vi "WildBugChilGru.vi"() -> ()   [LabVIEW 2014]
uses:
  <vilib>/Utility/miscctls.llb/LVPointTypeDef.ctl
  <vilib>/Utility/miscctls.llb/LVBoundsTypeDef.ctl
  <vilib>/Utility/miscctls.llb/LVPositionTypeDef.ctl
  <vilib>/Utility/xml.llb/Read From XML File(string).vi
  <vilib>/Utility/xml.llb/Write to XML File(string).vi
  <vilib>/Instr/_visa.llb/VISA Configure Serial Port (Instr).vi
  <vilib>/Analysis/3filter.llb/IIR Filter (DBL).vi
  <vilib>/gmath/NI_Gmath.lvlib
  <vilib>/Analysis/NI_AALBase.lvlib
panel:
  out "XY-Graph":cluster{dbl[], dbl[]}[](graph)
  in  "Registerkarte":T1(tab)
  in  "Zündung [Imp/U]":dbl=1.0
  in  "Übersetzung ermitteln aus":T2(ring)
  in  "Getriebe [1:]":dbl=4.0
  in  "Reifenumfang [m]":dbl=1.2
  in  "Dauer [s]":dbl=5.0
  in  "nKuWe/nRolle":dbl=1.0 format="%#.3f"
  in  "Lufttemperatur [°C]":dbl
  in  "Luftfeuchtigkeit [%]":dbl=43.8
  in  "Luftdruck [mbar]":dbl=1013.45
  in  "Messung Klimadaten":bool=TRUE
  in  "Gleitender Mittelwert":u8=35
  in  "Differenzenquotient":u8=12
  in  "n vom Gas [1/min]":dbl=5000.0
  in  "Rollengeber [Inkr/U]":u16=200
  in  "Rollenumfang [m]":dbl=0.613
  in  "Rollenträgheit [kgm²]":dbl=0.402
  in  "Recalc":bool
  in  "Leistung":bool=TRUE caption="Messung Klimadaten"
  in  "Ende":bool
  out "Datenspeicher":T3={"Fahrzeugdaten"="", "date/time string"="", "Rolle [Inkr/U]"=200, "Rollenumfang [m]"=0.613, "Rollenträgheit [kgm²]"=0.402, "Zündung [Imp/U]"=1.0, "Getriebe [1:]"=4.0, "Reifenumfang [m] "=1.2, "element"=0.0, "Gl. Mittelwert"=35, "Differenzenquotient"=12, "Polynom"=0, "dT [s]"=0.0, "element"=0.0, "Lufttemperatur [°C]"=0.0, "Luftfeuchtigkeit [%]"=43.8, "Luftdruck [mbar]"=1013.45, [], [], "Best Polynomial Fit"=[], [], "Übersetzung ermitteln aus"=0, "[s]"=5.0, "nmin [1/min]"=0.0, "nmax [1/min]"=0.0, "n vom Gas [1/min]"=5000.0, "dT-Array [s]"=[], [], "Boolesch"=TRUE, "Serielle Schnittstelle"="COM6", "nKuWe/nRolle"=1.0}
  out "COM-Fehlerrate":string="0 / 0,0%"
  in  "Konfiguration:":bool
  in  "Speichern":bool
  in  "Drucken":bool
  out "Pmax":string="0,0 PS"
  out "Ergebnis":string
  in  "Fahrzeugdaten":string
  out "Untersetzung\nermittelt":bool
  out "Untersetzung":dbl format="%#.3f"
  in  "Start":bool
  out "Füllstand Lesepuffer":u64(slide)=1 scale=1.0..100.0
  out "Hinterrad\n[km/h]":dbl(knob) step=5.0 scale=0.0..150.0
  out "Welle\n[1/min]":cluster{dbl, dbl}(knob) scale=0.0..14000.0
  out "Lesepuffer":string="\n"
  in  "Serielle Schnittstelle":refnum<visa-resource-name>="COM6"
  out "Untersetzung-Graph":dbl(graph)=198.99999999999997 caption="Untersetzung"
  # "1. n konstant halten\n2. START\n3. n weiter halten\n4. bei GO: Vollgas\n5. vom Gas gehen"
  # "Live-Tacho"
  # "Zündung\nRolle"
  # "Untersetzung aus:"
  # "Eingabe <> Messen"
  # "Tacho <> Leistung"
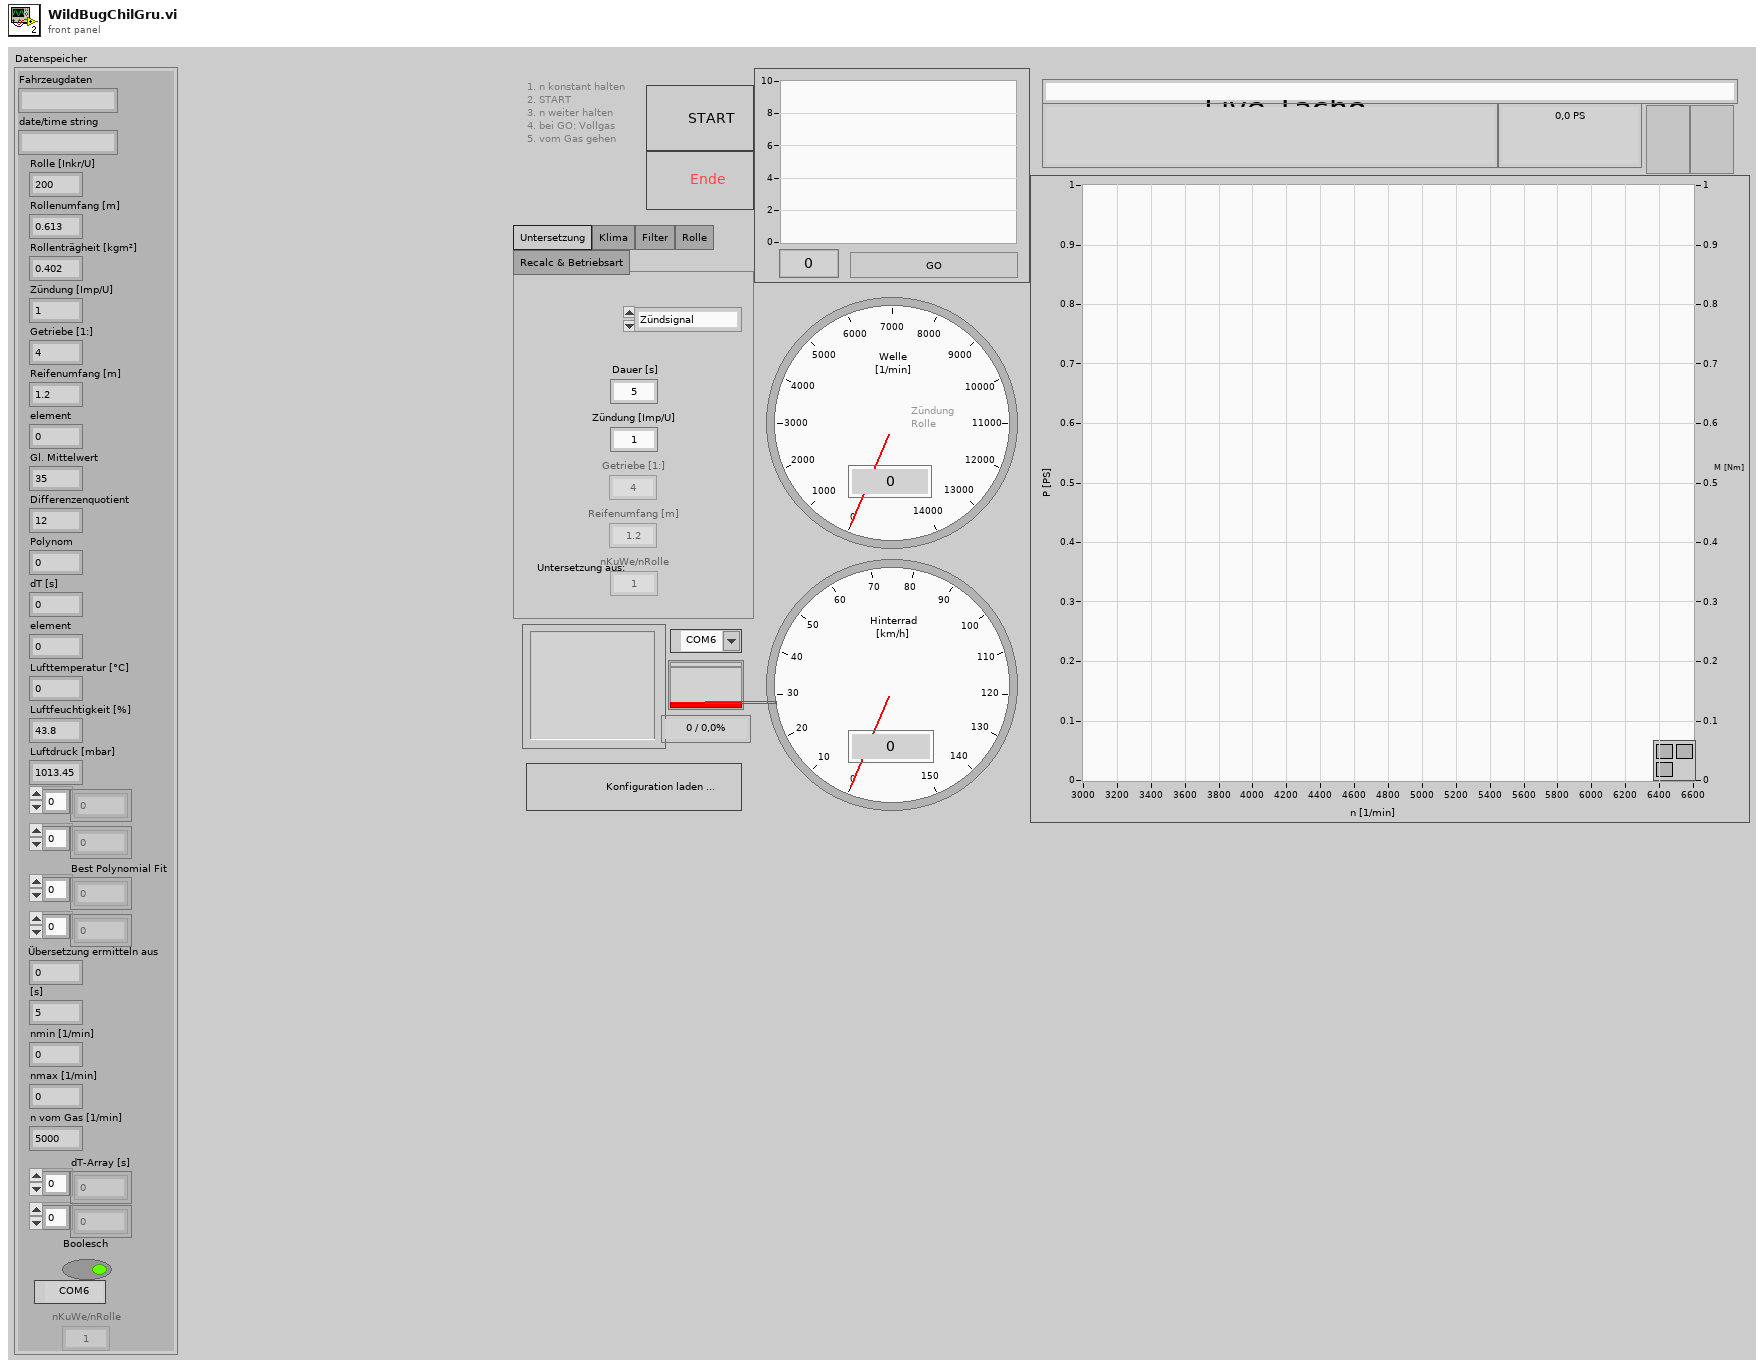
[diagram p1: front panel]
types:
  T1 = enum32{"Untersetzung", "Klima", "Filter", "Rolle", "Recalc & Betriebsart"}
  T2 = enum8{"Zündsignal", "Getriebe & Reifen", "nKuWe / nRolle"}
  T3 = cluster{"Fahrzeugdaten":string, "date/time string":string, "Rolle [Inkr/U]":u16, "Rollenumfang [m]":dbl, "Rollenträgheit [kgm²]":dbl, "Zündung [Imp/U]":dbl, "Getriebe [1:]":dbl, "Reifenumfang [m] ":dbl, "element":dbl, "Gl. Mittelwert":u8, "Differenzenquotient":u8, "Polynom":u8, "dT [s]":dbl, "element":dbl, "Lufttemperatur [°C]":dbl, "Luftfeuchtigkeit [%]":dbl, "Luftdruck [mbar]":dbl, dbl[], dbl[], "Best Polynomial Fit":dbl[], dbl[], "Übersetzung ermitteln aus":u8, "[s]":dbl, "nmin [1/min]":dbl, "nmax [1/min]":dbl, "n vom Gas [1/min]":dbl, "dT-Array [s]":dbl[], i32[], "Boolesch":bool, "Serielle Schnittstelle":refnum<visa-resource-name>, "nKuWe/nRolle":dbl}
  T4 = enum8{"Enabled", "Disabled", "Disabled and Grayed Out"}
  T5 = cluster{"Fahrzeugdaten":string, "date/time string":string, "Rollengeber [Inkr/U]":u16, "Rollenumfang [m]":dbl, "Rollenträgheit [kgm²]":dbl, "Zündung [Imp/U]":dbl, "Getriebe [1:]":dbl, "Reifenumfang [m] ":dbl, "mean value":dbl, "Gleitender Mittelwert":u8, "Differenzenquotient":u8, i32, dbl, "element":dbl, "Lufttemperatur [°C]":dbl, "Luftfeuchtigkeit [%]":dbl, "Luftdruck [mbar]":dbl, dbl[], dbl[], dbl[], dbl[], "Übersetzung ermitteln aus":enum8{"Zündsignal", "Getriebe & Reifen", "nKuWe / nRolle"}, "Dauer [s]":dbl, dbl, dbl, "n vom Gas [1/min]":dbl, dbl[], i32[], "Messung Klimadaten":bool, "VISA resource name out":refnum<visa-resource-name>, "nKuWe/nRolle":dbl}
  T6 = cluster{"Fahrzeugdaten":string, "date/time string":string, "Rolle [Inkr/U]":u16, "Rollenumfang [m]":dbl, "Rollenträgheit [kgm²]":dbl, "Zündung [Imp/U]":dbl, "Getriebe [1:]":dbl, "Reifenumfang [m] ":dbl, "element":dbl, "Gl. Mittelwert":u8, "Differenzenquotient":u8, "Polynom":u8, "element":dbl, "element":dbl, "Lufttemperatur [°C]":dbl, "Luftfeuchtigkeit [%]":dbl, "Luftdruck [mbar]":dbl, dbl[], dbl[], "Best Polynomial Fit":dbl[], dbl[], "Übersetzung ermitteln aus":u8, "[s]":dbl, "nmin [1/min]":dbl, "nmax [1/min]":dbl, "n vom Gas [1/min]":dbl, dbl[], i32[], "Boolesch":bool, "Serielle Schnittstelle":refnum<visa-resource-name>, dbl}
  T7 = typedef "LVPointTypeDef.ctl" = cluster{"Horizontal":i16, "Vertical":i16}
  T8 = typedef "LVPositionTypeDef.ctl" = cluster{"Left":i32, "Top":i32}
  T9 = typedef "LVBoundsTypeDef.ctl" = cluster{"Width":u32, "Height":u32}
  T10 = enum16{"Left Button", "Center Button", "Right Button", "Window Close"}
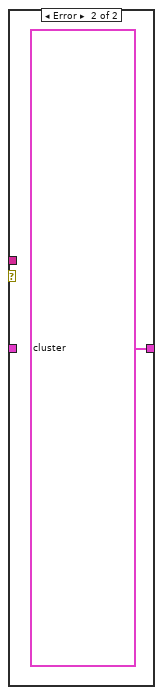
[diagram p2: hidden frame]
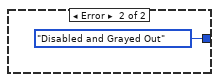
[diagram p3: hidden frame]
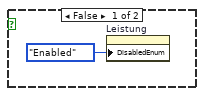
[diagram p4: hidden frame]
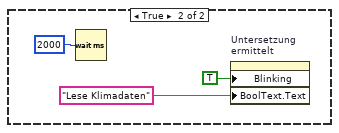
[diagram p5: hidden frame]
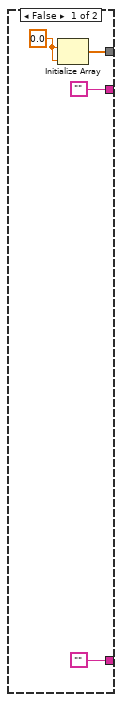
[diagram p8: hidden frame]
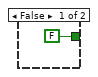
[diagram p9: hidden frame]
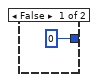
[diagram p11: hidden frame]
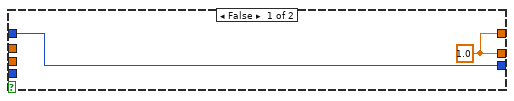
[diagram p13: hidden frame]
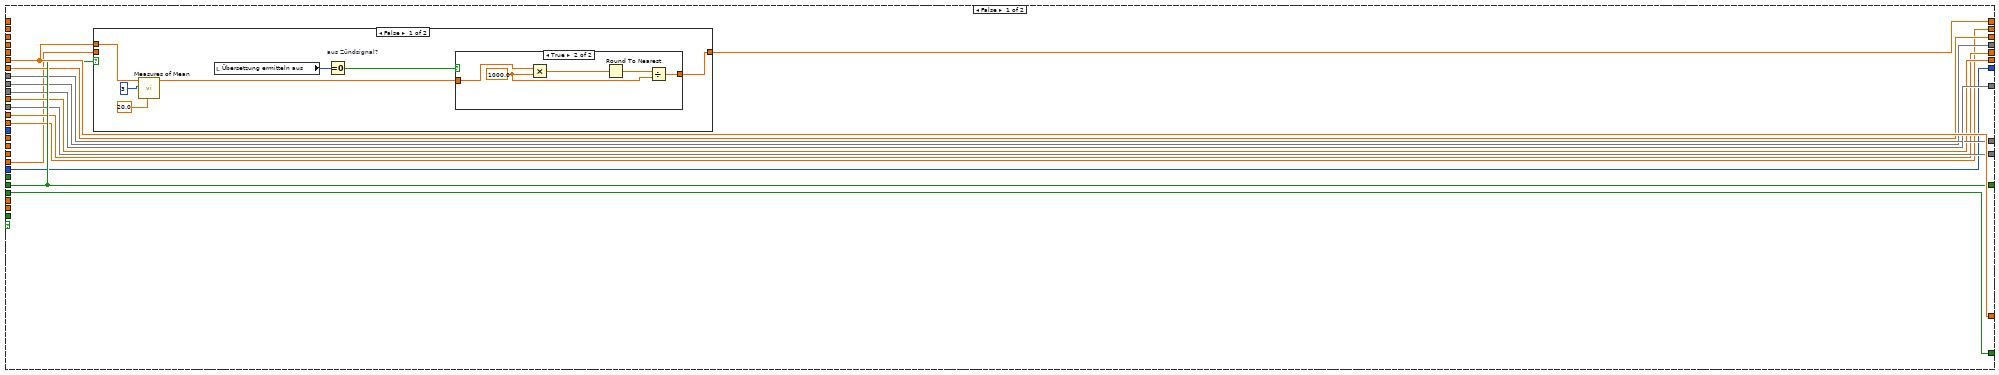
[diagram p14: hidden frame]
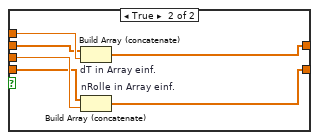
[diagram p17: hidden frame]
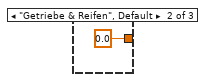
[diagram p20: hidden frame]
diagram:
  n1 = while {
    stop <- w1 stop-if-true
    n2 = local read "Start"() -> (w2:bool)
    n3 = case shown="True" w2 {
      frame False {
        n4 = property on="Leistung" class="Bool. (strikt)"("DisabledEnum"=T4."Enabled" ("Deaktiviert")) -> ()  [unwired: 2 in, 2 out]
      }
      frame True {
        n5 = flat-sequence {
          tunnel: [w137] -> w123
          tunnel: [w136] -> w122
          tunnel: [w134] -> w121
          tunnel: ["Leistung"] -> w8
          tunnel: w123 -> [w148]
          tunnel: w122 -> [w152]
          tunnel: [0] -> w120
          tunnel: [1.0 ("element")] -> w119
          tunnel: [w150] -> w118
          tunnel: [w162] -> w117
          tunnel: [0] -> w116
          tunnel: [w150] -> w115
          tunnel: [-5] -> w114
          tunnel: [w159] -> w113
          tunnel: [w157] -> w112
          tunnel: [w156] -> w111
          tunnel: [0.0] -> w110
          tunnel: [w148] -> w109
          tunnel: [w152] -> w108
          tunnel: w121 -> [w151]
          tunnel: [w151] -> w107
          tunnel: w8 -> [w147]
          tunnel: [w147] -> w4
          tunnel: w120 -> [w189]
          tunnel: [w189] -> w106
          tunnel: w119 -> [w188]
          tunnel: [w188] -> w105
          tunnel: w118 -> [w187]
          tunnel: [w187] -> w104
          tunnel: w117 -> [w186]
          tunnel: [w186] -> w103
          tunnel: w116 -> [w185]
          tunnel: [w185] -> w102
          tunnel: w115 -> [w184]
          tunnel: [w184] -> w101
          tunnel: w114 -> [w183]
          tunnel: [w183] -> w100
          tunnel: w113 -> [w182]
          tunnel: [w182] -> w99
          tunnel: w112 -> [w181]
          tunnel: [w181] -> w98
          tunnel: w111 -> [w180]
          tunnel: [w180] -> w97
          tunnel: w110 -> [w179]
          tunnel: [w179] -> w96
          tunnel: w109 -> [w178]
          tunnel: [w175] -> w95
          tunnel: w108 -> [w177]
          tunnel: [w176] -> w94
          tunnel: w107 -> [w174]
          tunnel: [w174] -> w10
          tunnel: [w173] -> w5
          tunnel: w4 -> [w173]
          tunnel: w106 -> [w214]
          tunnel: [w214] -> w93
          tunnel: w105 -> [w213]
          tunnel: [w213] -> w92
          tunnel: w104 -> [w212]
          tunnel: [w212] -> w91
          tunnel: w103 -> [w211]
          tunnel: [w211] -> w90
          tunnel: w102 -> [w210]
          tunnel: [w210] -> w89
          tunnel: w101 -> [w209]
          tunnel: [w209] -> w88
          tunnel: w100 -> [w208]
          tunnel: [w208] -> w87
          tunnel: w99 -> [w207]
          tunnel: [w207] -> w86
          tunnel: w98 -> [w206]
          tunnel: [w206] -> w85
          tunnel: w97 -> [w205]
          tunnel: [w205] -> w84
          tunnel: w96 -> [w204]
          tunnel: [w204] -> w83
          tunnel: w95 -> [w203]
          tunnel: [w203] -> w82
          tunnel: w94 -> [w202]
          tunnel: [w202] -> w81
          tunnel: [w200] -> w11
          tunnel: w10 -> [w200]
          tunnel: [w199] -> w6
          tunnel: w5 -> [w199]
          tunnel: w93 -> [w231]
          tunnel: [w231] -> w80
          tunnel: w92 -> [w230]
          tunnel: [w230] -> w79
          tunnel: w91 -> [w229]
          tunnel: [w229] -> w78
          tunnel: w90 -> [w228]
          tunnel: [w228] -> w77
          tunnel: w89 -> [w227]
          tunnel: [w227] -> w76
          tunnel: w88 -> [w226]
          tunnel: [w226] -> w75
          tunnel: w87 -> [w225]
          tunnel: [w225] -> w74
          tunnel: w86 -> [w224]
          tunnel: [w224] -> w73
          tunnel: w85 -> [w223]
          tunnel: [w223] -> w72
          tunnel: w84 -> [w222]
          tunnel: [w222] -> w71
          tunnel: w83 -> [w221]
          tunnel: [w221] -> w70
          tunnel: w82 -> [w220]
          tunnel: [w219] -> w69
          tunnel: w81 -> [w217]
          tunnel: [w218] -> w68
          tunnel: w11 -> [w216]
          tunnel: [w215] -> w7
          tunnel: w6 -> [w215]
          tunnel: w80 -> [w296]
          tunnel: w79 -> [w295]
          tunnel: w78 -> [w294]
          tunnel: w77 -> [w293]
          tunnel: w76 -> [w292]
          tunnel: w75 -> [w291]
          tunnel: w74 -> [w290]
          tunnel: w73 -> [w289]
          tunnel: w72 -> [w288]
          tunnel: w71 -> [w287]
          tunnel: w70 -> [w286]
          tunnel: w69 -> [w267]
          tunnel: [w296] -> w67
          tunnel: [w295] -> w66
          tunnel: [w294] -> w65
          tunnel: [w293] -> w64
          tunnel: [w292] -> w63
          tunnel: [w291] -> w62
          tunnel: [w290] -> w61
          tunnel: [w289] -> w60
          tunnel: [w288] -> w59
          tunnel: [w287] -> w58
          tunnel: [w286] -> w57
          tunnel: [w267] -> w56
          tunnel: [w266] -> w55
          tunnel: [w285] -> w54
          tunnel: [w284] -> w53
          tunnel: [w283] -> w52
          tunnel: ["Gleitender Mittelwert"] -> w51
          tunnel: w68 -> [w266]
          tunnel: [w261] -> w14
          tunnel: [w260] -> w13
          tunnel: [w259] -> w9
          tunnel: w7 -> [w259]
          tunnel: [w305] -> w23
          tunnel: [w306] -> w24
          tunnel: [w307] -> w25
          tunnel: [w308] -> w26
          tunnel: [w299] -> w21
          tunnel: [w298] -> w22
          tunnel: [w309] -> w27
          tunnel: [w310] -> w28
          tunnel: [w311] -> w30
          tunnel: [w312] -> _
          tunnel: [w313] -> w32
          tunnel: [w314] -> w33
          tunnel: [w315] -> w46
          tunnel: [w316] -> w12
          tunnel: [w317] -> w48
          tunnel: [w318] -> w49
          tunnel: [w319] -> w50
          tunnel: w67 -> [w319]
          tunnel: w66 -> [w318]
          tunnel: w65 -> [w317]
          tunnel: w64 -> [w316]
          tunnel: w63 -> [w315]
          tunnel: w62 -> [w314]
          tunnel: w61 -> [w313]
          tunnel: w60 -> [w312]
          tunnel: w59 -> [w311]
          tunnel: w58 -> [w310]
          tunnel: w57 -> [w309]
          tunnel: w56 -> [w301]
          tunnel: w55 -> [w300]
          tunnel: w54 -> [w308]
          tunnel: w53 -> [w307]
          tunnel: w52 -> [w306]
          tunnel: w51 -> [w305]
          frame #0 {
            w142 = u16 0 items=["None", "XON/XOFF", "RTS/CTS", "XON/XOFF & RTS/CTS", "DTR/DSR", "XON/XOFF & DTR/DSR"] ("flow control (0:none)")
            w143 = u16 10 items=["1.0"=10, "1.5"=15, "2.0"=20] ("stop bits (10: 1 bit)")
            w135 = FALSE  # Enable Termination Char (T)
            w138 = u32 10000  # timeout (10sec)
            n6 = call-poly "VISA Configure Serial Port"("VISA resource name"="Serielle Schnittstelle", "timeout (10sec)"=w138, "Enable Termination\nChar (T)"=w135, "baud rate (9600)"=u32 115200 ("baudrate (250000)"), "data bits (8)"=u16 8, "parity (0:none)"=enum16{"None", "Odd", "Even", "Mark", "Space"}."None", "stop bits (10: 1 bit)"=w143, "flow control (0:none)"=w142) -> ("VISA resource name out"=w140:refnum<visa-resource-name>, "error out"=w139:errorcluster)  [unwired: 6 in]
            n7 = And(x="Messung Klimadaten", y="Leistung") -> (x .and. y?=w134:bool)
            n8 = VISA Clear(VISA resource name=w140, error in (no error)=w139) -> (VISA resource name out=w137:refnum<visa-resource-name>, error out=w136:errorcluster)
          }
          frame #1 {
            w149 = T4."Disabled and Grayed Out" ("Deaktiviert")
            w155 = 0.0  # Graphen löschen
            w158 = 0
            w163 = 0.0
            w150 = FALSE
            w156 = ""
            n9 = case shown="False" w151 {
              frame False {
                n10 = property on="Untersetzung\nermittelt" class="Bool. (strikt)"("Blinking"=TRUE ("Blinkend"), "BoolText.Text"="Initialisiere" ("Beschriftung.Text")) -> ()  [unwired: 2 in, 2 out]
              }
              frame True {
                n11 = Wait (ms)(milliseconds to wait=u32 2000 ("Zu wartende ms")) -> ()  [unwired: 1 out]
                n12 = property on="Untersetzung\nermittelt" class="Bool. (strikt)"("Blinking"=TRUE ("Blinkend"), "BoolText.Text"="Lese Klimadaten" ("Beschriftung.Text")) -> ()  [unwired: 2 in, 2 out]
              }
            }
            n13 = Build Array(w155) -> (w154:dbl[])
            n14 = property on="Drucken" class="Bool. (strikt)"("DisabledEnum"=w149) -> ()  [unwired: 2 in, 2 out]
            n15 = property on="Übersetzung ermitteln aus" class="Enum (strikt)"("DisabledEnum"=w149) -> ()  [unwired: 2 in, 2 out]
            n16 = property on="Konfiguration:" class="Bool. (strikt)"("DisabledEnum"=w149) -> ()  [unwired: 2 in, 2 out]
            n17 = property on="Ende" class="Bool. (strikt)"("DisabledEnum"=w149) -> ()  [unwired: 2 in, 2 out]
            n18 = property on="Leistung" class="Bool. (strikt)"("DisabledEnum"=w149) -> ()  [unwired: 2 in, 2 out]
            n19 = property on="Speichern" class="Bool. (strikt)"("DisabledEnum"=w149) -> ()  [unwired: 2 in, 2 out]
            n20 = property on="Untersetzung-Graph" class="SVDiagr (strikt)"("History Data"=w154) -> ()  [unwired: 2 in, 2 out]
            n21 = local write "Pmax"(w156) -> ()
            n22 = local write "COM-Fehlerrate"(w156) -> ()
            n23 = local write "Ergebnis"(w156) -> ()
            n24 = Initialize Array(w158, w158) -> (w157:i32[])
            n25 = Initialize Array(w163, w163) -> (w162:dbl[])
            n26 = Initialize Array(0.0 ("y"), 0) -> (w159:dbl[])
          }
          frame #2 {
            n27 = case shown="True" w174 {
              tunnel: w178 -> [w191 w195]
              tunnel: w177 -> [w190 w194]
              tunnel: [w190 w193] -> w176
              tunnel: [w191 w192] -> w175
              frame False {
              }
              frame True {
                n28 = Concatenate Strings("e" ("String"), "\n") -> (w198:string)
                n29 = VISA Write(VISA resource name=w195, write buffer=w198, error in (no error)=w194) -> (VISA resource name out=w192:refnum<visa-resource-name>, error out=w193:errorcluster)  [unwired: 1 out]
              }
            }
          }
          frame #3 {
            n30 = Wait (ms)(milliseconds to wait=u32 500 ("Zu wartende ms")) -> ()  [unwired: 1 out]
          }
          frame #4 {
            n31 = case shown="True" w216 {
              tunnel: w220 -> [w233 w254]
              tunnel: [w233 w253] -> w219
              tunnel: [w232 w252] -> w218
              tunnel: w217 -> [w232 w251]
              frame False {
              }
              frame True {
                w236 = ";" ("Regulärer Ausdruck")
                n32 = property class="Instr"(reference=w254, error in=w251) -> (reference out=w257:refnum<visa-resource-name>, error out=w256:errorcluster, "Serial Settings:Number of Bytes at Serial Port"=w255:u32)
                n33 = VISA Read(VISA resource name=w257, byte count=w255, error in (no error)=w256) -> (VISA resource name out=w253:refnum<visa-resource-name>, read buffer=w248:string, error out=w252:errorcluster)  [unwired: 1 out]
                n34 = Search and Replace String(replace all?=TRUE ("Alle ersetzen? (F)"), input string=w248, search string="." ("Such-String"), replace string="," ("Ersetzungs-String (\"\")")) -> (result string=w241:string)  [unwired: 4 in, 3 out]
                n35 = Match Pattern(string=w241, regular expression=w236) -> (before substring=w239:string, after substring=w240:string)  [unwired: 1 in, 2 out]
                n36 = Match Pattern(string=w240, regular expression=w236) -> (before substring=w238:string, after substring=w237:string)  [unwired: 1 in, 2 out]
                n37 = Fract/Exp String To Number(string=w239, offset=0 ("Offset")) -> (number=w247:dbl)  [unwired: 2 in, 1 out]
                n38 = local write "Lufttemperatur [°C]"(w247) -> ()
                n39 = Fract/Exp String To Number(string=w238) -> (number=w244:dbl)  [unwired: 3 in, 1 out]
                n40 = Match Pattern(string=w237, regular expression=w236) -> (before substring=w235:string)  [unwired: 1 in, 3 out]
                n41 = Fract/Exp String To Number(string=w235) -> (number=w246:dbl)  [unwired: 3 in, 1 out]
                n42 = Divide(x=w244, y=100.0 ("x")) -> (x/y=w245:dbl)
                n43 = local write "Luftdruck [mbar]"(w245) -> ()
                n44 = local write "Luftfeuchtigkeit [%]"(w246) -> ()
              }
            }
          }
          frame #5 {
            n45 = Wait (ms)(milliseconds to wait=u32 2000 ("Zu wartende ms")) -> ()  [unwired: 1 out]
            n46 = Add(x="Lufttemperatur [°C]", y=273.15) -> (x+y=w279:dbl)
            n47 = Divide ("M_Welle [Nm]")(x=w279, y=293.15) -> (x/y=w277:dbl)
            n48 = Power Of X(1:w277, 2:0.5) -> (0:w274:dbl)
            n49 = Divide ("M_Welle [Nm]")(x=1013.0, y="Luftdruck [mbar]") -> (x/y=w275:dbl)
            n50 = Multiply "Korrekturfaktor DIN 70020"(x=w275, y=w274) -> (x*y=w285:dbl)
            n51 = local read "Differenzenquotient"() -> (w262:u8)
            n52 = Divide(x="Gleitender Mittelwert", y=2) -> (x/y=w271:dbl)
            n53 = Round Toward -Infinity(1:w271) -> (0:w270:dbl)
            n54 = call <vilib>:"Smoothing Filter Coefficients.vi"("shape"=1, "half-width"=w270, "type"=0) -> ("forward coefficients"=w283:dbl[], "reverse coefficients"=w284:dbl[])  [unwired: 6 in, 1 out]
            n55 = call <vilib>:"Smoothing Filter Coefficients.vi"("shape"=0, "half-width"=w262, "type"=0) -> ("forward coefficients"=w260:dbl[], "reverse coefficients"=w261:dbl[])  [unwired: 6 in, 1 out]
          }
          frame #6 {
            n56 = Concatenate Strings("m" ("String"), "\n") -> (w304:string)
            n57 = property on="Untersetzung\nermittelt" class="Bool. (strikt)"("Blinking"=FALSE ("Blinkend")) -> ()  [unwired: 2 in, 2 out]
            n58 = VISA Write(VISA resource name=w301, write buffer=w304, error in (no error)=w300) -> (VISA resource name out=w298:refnum<visa-resource-name>, error out=w299:errorcluster)  [unwired: 1 out]
          }
        }
        n59 = while {
          tunnel: w22 -> [w440]
          tunnel: w21 -> [w439]
          shift-right: [w506] -> _
          shift-left: w28 -> [w455]
          shift-right: [w501] -> _
          shift-left: w27 -> [w505]
          shift-right: [w500] -> _
          shift-left: w27 -> [w504]
          shift-right: [w459] -> _
          shift-left: w27 -> [w503]
          shift-right: [w485] -> _
          shift-left: w50 -> [w502]
          shift-right: [w447] -> w35
          shift-left: w49 -> [_]
          shift-right: [w464] -> w39
          shift-left: w27 -> [w434]
          shift-right: [w429] -> w37
          shift-left: w27 -> [w461]
          shift-right: [w460] -> _
          shift-left: w12 -> [w497]
          shift-right: [w432] -> _
          shift-left: w48 -> [w474]
          shift-right: [w441] -> _
          shift-left: w12 -> [_]
          shift-right: [w446] -> _
          shift-left: w12 -> [_]
          shift-right: [w494] -> w38
          shift-left: w12 -> [w492]
          shift-right: [w493] -> _
          shift-left: w12 -> [w491]
          shift-right: [w480] -> w45
          shift-left: w12 -> [w490]
          shift-right: [w484] -> _
          shift-left: w12 -> [w488]
          shift-right: [w483] -> w15
          shift-left: w12 -> [w489]
          shift-right: [w482] -> w44
          shift-left: w12 -> [w487]
          shift-right: [w481] -> w43
          shift-left: w12 -> [w486]
          tunnel: [w479] -> w47
          shift-right: [w475] -> w42
          shift-left: w46 -> [w477]
          tunnel: [w478] -> w18
          tunnel: ["n vom Gas [1/min]"] -> w41
          tunnel: ["Rollenumfang [m]"] -> w40
          tunnel: ["Rollenumfang [m]"] -> w34
          shift-right: [w471] -> _
          shift-left: w33 -> [w438]
          shift-right: [w465] -> _
          shift-left: w32 -> [w470]
          shift-right: [w466] -> _
          shift-left: w27 -> [w469]
          shift-right: [w467] -> _
          shift-left: w27 -> [w468]
          shift-right: [w437] -> w31
          shift-left: w12 -> [w463]
          shift-right: [w458] -> _
          shift-left: _ -> [w457]
          shift-right: [w462] -> w29
          shift-left: w30 -> [w456]
          tunnel: [w454] -> w19
          tunnel: w26 -> [w447]
          tunnel: w25 -> [w441]
          tunnel: w24 -> [w446]
          tunnel: w23 -> [w445]
          tunnel: w14 -> [w436]
          tunnel: w13 -> [w435]
          tunnel: w9 -> [w428]
          stop <- w479 stop-if-true
          n60 = property class="Instr"(reference=w440, error in=w439) -> (reference out=w450:refnum<visa-resource-name>, error out=w449:errorcluster, "Serial Settings:Number of Bytes at Serial Port"=w452:u32)
          n61 = Greater?(x=w452, y=u32 1 ("min. Bytes")) -> (0:w448:bool)
          n62 = case shown="True" w448 {
            tunnel: w452 -> [_ w512]
            tunnel: [u32 0 ("Bytes at Port") w512] -> w451
            frame False {
            }
            frame True {
            }
          }
          n63 = case shown="1.." w451 {
            selector: w451 -> [_ w798]
            tunnel: [w748 w792] -> w478
            tunnel: [w747 w793] -> w454
            tunnel: [w752 w794] -> w500
            tunnel: [w753 w791] -> w501
            tunnel: w455 -> [w754 w789]
            tunnel: [w754 w787] -> w506
            tunnel: w505 -> [w753 w779]
            tunnel: w504 -> [w752 w778]
            tunnel: [w749 w777] -> w459
            tunnel: w503 -> [w749 w776]
            tunnel: w502 -> [w751 _]
            tunnel: [w751 w759] -> w485
            tunnel: [w750 w765] -> w458
            tunnel: w457 -> [w750 w764]
            tunnel: w450 -> [w747 w756]
            tunnel: w449 -> [w748 w755]
            frame 0, Default {
              # "No data in from serial port - Nothing to do."
            }
            frame 1.. {
              # "Hz Drum"
              n64 = VISA Read(VISA resource name=w756, byte count=w798, error in (no error)=w755) -> (VISA resource name out=w793:refnum<visa-resource-name>, read buffer=w790:string, error out=w792:errorcluster)  [unwired: 1 out]
              n65 = Concatenate Strings(w789, w790) -> (w761:string)
              "Lesepuffer" <- w761
              n66 = Spreadsheet String To Array(delimiter (Tab)="\n" ("regular expression"), format string="%s" ("regular expression"), spreadsheet string=w761, array type (2D Dbl)=string[] [] ("Array 2")) -> (array=w770:string[])
              n67 = Match Pattern(string=w761, regular expression="[\\n]") -> (before substring=w768:string, after substring=w788:string, offset past match=w802:i32)  [unwired: 1 in, 1 out]
              n68 = Array Size(array=w770) -> (size(s)=w774:i32)
              n69 = Match Pattern(string=w768, regular expression="[;]") -> (before substring=w766:string, after substring=w767:string, offset past match=w763:i32)  [unwired: 1 in, 1 out]
              n70 = Subtract "aktuelle Zeilenanzahl"(x=w774, y=1) -> (x-y=w759:i32)
              n71 = property on="Füllstand Lesepuffer" class="Schieber (strikt)"() -> ("Scale.Maximum"=w758:dbl)  [unwired: 2 in, 2 out]
              n72 = Match Pattern(string=w767, regular expression="[;]") -> (before substring=w797:string, after substring=w800:string, offset past match=w785:i32)  [unwired: 1 in, 1 out]
              n73 = Match Pattern(string=w800, regular expression="[;]") -> (before substring=w796:string, after substring=w795:string, offset past match=w783:i32)  [unwired: 1 in, 1 out]
              n74 = Greater Or Equal To 0?(x=w763) -> (x >= 0?=w762:bool)
              n75 = Greater?(x=w759, y=w758) -> (0:w760:bool)
              n76 = Greater Or Equal To 0?(x=w783) -> (x >= 0?=w782:bool)
              n77 = Greater Or Equal To 0?(x=w785) -> (x >= 0?=w784:bool)
              n78 = Greater Or Equal To 0?(x=w802) -> (x >= 0?=w786:bool)
              n79 = Select(t=w759, s=w760, f=w758) -> (s? t:f=w757:dbl)
              n80 = Build Array(w786, w784, w762, w782) -> (w781:bool[])
              n81 = property on="Füllstand Lesepuffer" class="Schieber (strikt)"("Scale.Maximum"=w757) -> ()  [unwired: 2 in, 2 out]
              n82 = And Array Elements(Boolean array=w781) -> (logical AND=w780:bool)
              n83 = case shown="True" w780 {
                tunnel: w797 -> [_ w813]
                tunnel: w796 -> [_ w818]
                tunnel: w795 -> [_ w817]
                tunnel: [w806 w816] -> w794
                tunnel: [w807 w815] -> w791
                tunnel: w788 -> [_ w814]
                tunnel: [w808 w814] -> w787
                tunnel: w761 -> [w808 _]
                tunnel: w779 -> [w807 _]
                tunnel: w778 -> [w806 _]
                tunnel: [w805 w812] -> w777
                tunnel: w776 -> [w805 _]
                tunnel: w766 -> [_ w811]
                tunnel: [w804 w809] -> w765
                tunnel: w764 -> [w804 _]
                frame False {
                }
                frame True {
                  # "Cyclecounter"
                  # "Hz ComLevel"
                  # "ComLevel\nLevel 10 =   6Hz \nLevel 5 =   12Hz \nLevel 4 =   15Hz\nLevel 3 =   20Hz\nLevel 2 =   33Hz\nLevel 1 =   62Hz"
                  # "Hz Drum"
                  # "Hz Engine"
                  # "t4m"
                  n84 = Fract/Exp String To Number(string=w811) -> (number=w810:dbl)  [unwired: 3 in, 1 out]
                  n85 = Fract/Exp String To Number(string=w817) -> (number=w816:dbl)  [unwired: 3 in, 1 out]
                  n86 = Fract/Exp String To Number(string=w813) -> (number=w812:dbl)  [unwired: 3 in, 1 out]
                  n87 = To Long Integer(number=w810) -> (32bit integer=w809:i32)
                  n88 = Fract/Exp String To Number(string=w818) -> (number=w815:dbl)  [unwired: 3 in, 1 out]
                }
              }
            }
          }
          "Füllstand Lesepuffer" <- w485
          n89 = Not Equal?(x=w457, y=w458) -> (x != y?=w442:bool)
          n90 = case shown="True" w442 {
            tunnel: w470 -> [w516 w527]
            tunnel: [w516 w539] -> w465
            tunnel: w469 -> [w515 w538]
            tunnel: [w515 w524] -> w466
            tunnel: w468 -> [w514 w537]
            tunnel: [w514 w525] -> w467
            tunnel: w458 -> [_ w523]
            tunnel: w456 -> [w513 w522]
            tunnel: [w513 w526] -> w462
            frame False {
            }
            frame True {
              n91 = Build Array (concatenate)(w522, w523) -> (w526:i32[])
              n92 = Greater Or Equal To 0?(x=w527) -> (x >= 0?=w528:bool)
              n93 = case shown="True" w528 {
                tunnel: [w540 w551] -> w524
                tunnel: [w540 w552] -> w525
                tunnel: [w541 w543] -> w539
                tunnel: w538 -> [_ w545]
                tunnel: w537 -> [_ w553]
                tunnel: w523 -> [w541 w542]
                tunnel: w527 -> [_ w543]
                frame False {
                  w540 = 1.0
                }
                frame True {
                  w549 = 65536.0
                  n94 = Add(x=w543, y=w545) -> (x+y=w544:dbl)
                  n95 = Divide(x=w544, y=w549) -> (x/y=w554:dbl)
                  n96 = Increment(x=w553) -> (x+1=w552:dbl)
                  n97 = Round Toward -Infinity(1:w554) -> (0:w550:dbl)
                  n98 = Multiply(x=w550, y=w549) -> (x*y=w548:dbl)
                  n99 = Add(x=w548, y=w542) -> (x+y=w547:dbl)
                  n100 = Increment(x=w547) -> (x+1=w546:dbl)
                  n101 = Subtract(x=w546, y=w543) -> (x-y=w551:dbl)
                }
              }
              n102 = Subtract(x=w524, y=w525) -> (x-y=w519:dbl)
              n103 = Decrement(x=w519) -> (x-1=w518:dbl)
              n104 = Max & Min(x=0, y=w518) -> (max(x,y)=w517:dbl)  [unwired: 1 out]
              n105 = Divide(x=w517, y=w524) -> (x/y=w531:dbl)
              n106 = Greater Than 0?(x=w517) -> (x > 0?=w521:bool)
              n107 = Select(t=u32 16711680, s=w521, f=u32 0) -> (s? t:f=w532:u32)
              n108 = Multiply(x=w531, y=100.0) -> (x*y=w529:dbl)
              n109 = property on="COM-Fehlerrate" class="Str"("Text.TextColor"=w532) -> ()  [unwired: 2 in, 2 out]
              n110 = Format Into String(format string="%d / %.1f%%" ("Format-String"), w517, w529) -> (resulting string=→"COM-Fehlerrate":string)  [unwired: 2 in, 1 out]
            }
          }
          n111 = case "Case-Struktur" shown="True" w442 {
            tunnel: w501 -> [w728 w740]
            tunnel: w500 -> [w727 w739]
            tunnel: [w728 w738] -> w499
            tunnel: [w727 w737] -> w498
            tunnel: w459 -> [_ w732]
            tunnel: w434 -> [w726 _]
            tunnel: [w726 w731] -> w464
            tunnel: w461 -> [_ w736]
            tunnel: "Rollenumfang [m]" -> [_ w735]
            frame False {
            }
            frame True {
              w746 = 60.0 ("y")
              n112 = Reciprocal "Abtastzeit [s]"(x=w732) -> (1/x=w731:dbl)
              n113 = Divide "R [1/s]"(x=w739, y="Rollengeber [Inkr/U]") -> (x/y=w745:dbl)
              n114 = Divide(x=w740, y="Zündung [Imp/U]") -> (x/y=w743:dbl)
              n115 = Multiply "nZ gemessen [1/min]"(x=w743, y=w746) -> (x*y=w738:dbl)
              n116 = Multiply "nR [1/min]"(x=w746, y=w745) -> (x*y=w737:dbl)
              n117 = Multiply "nZ berechnet [1/min]"(x=w737, y=w736) -> (x*y=w744:dbl)
              n118 = Multiply "[m/min]"(x=w737, y=w735) -> (x*y=w741:dbl)
              n119 = Multiply "[km/h]"(x=w741, y=0.06) -> (x*y=→"Hinterrad\n[km/h]":dbl)
              n120 = Bundle(w738, w744) -> (→"Welle\n[1/min]":cluster{dbl, dbl})  [unwired: 1 in]
            }
          }
          n121 = case shown="True" w442 {
            tunnel: w499 -> [_ w647]
            tunnel: w498 -> [_ w646]
            tunnel: "Rollenumfang [m]" -> [_ w650]
            tunnel: [w566 w621] -> w429
            tunnel: w461 -> [w555 w621]
            tunnel: w474 -> [w567 w589]
            tunnel: w497 -> [w568 w653]
            tunnel: [w567 w613] -> w432
            tunnel: [w568 w652] -> w460
            tunnel: w441 -> [_ w649]
            tunnel: w446 -> [_ w648]
            tunnel: [w565 w585] -> w494
            tunnel: [w564 w593] -> w493
            tunnel: w492 -> [w565 w645]
            tunnel: w491 -> [w564 _]
            tunnel: w445 -> [_ w602]
            tunnel: [w563 w627] -> w480
            tunnel: w490 -> [w563 _]
            tunnel: [w562 w592] -> w484
            tunnel: w488 -> [w562 _]
            tunnel: [w561 w628] -> w483
            tunnel: w489 -> [w561 _]
            tunnel: [w560 w639] -> w482
            tunnel: w487 -> [w560 _]
            tunnel: [w559 w638] -> w481
            tunnel: w486 -> [w559 _]
            tunnel: w447 -> [_ w631]
            tunnel: w477 -> [w558 w626]
            tunnel: "n vom Gas [1/min]" -> [_ w615]
            tunnel: [w558 w625] -> w475
            tunnel: w474 -> [_ w624]
            tunnel: w438 -> [w557 w620]
            tunnel: [w557 w619] -> w471
            tunnel: w464 -> [_ w618]
            tunnel: [w556 w586] -> w437
            tunnel: w463 -> [w556 w617]
            tunnel: w436 -> [_ w600]
            tunnel: w435 -> [_ w599]
            tunnel: w428 -> [_ w583]
            frame False {
              n122 = case shown="False" w567 {
                tunnel: w568 -> [w575 _]
                tunnel: [w569 w582] -> w566
                tunnel: w555 -> [_ w582]
                frame False {
                  n123 = call <vilib>:"Measures of Mean.vi"("percent (trim)"=20.0, "type"=3, "x array"=w575) -> ("mean value"=w570:dbl)  [unwired: 7 in, 1 out]
                  n124 = local read "Übersetzung ermitteln aus"() -> (w572:T2)
                  n125 = Equal To 0? "aus Zündsignal?"(x=w572) -> (x = 0?=w571:bool)
                  n126 = case shown="True" w571 {
                    tunnel: w570 -> [w576 w581]
                    tunnel: [w576 w577] -> w569
                    frame False {
                    }
                    frame True {
                      w578 = 1000.0
                      n127 = Multiply(x=w581, y=w578) -> (x*y=w580:dbl)
                      n128 = Round To Nearest(number=w580) -> (nearest integer value=w579:dbl)
                      n129 = Divide(x=w579, y=w578) -> (x/y=w577:dbl)
                    }
                  }
                }
                frame True {
                }
              }
            }
            frame True {
              w634 = 0.00135962  # [W] in [PS]
              w641 = 0.10471975511965978  # 2*Pi/60
              n130 = Not(x=w589) -> (.not. x?=w588:bool)
              n131 = Or(x=w583, y=w588) -> (x .or. y?=w587:bool)
              n132 = local read "Übersetzung ermitteln aus"() -> (w590:T2)
              n133 = case shown="False" w587 {
                tunnel: w646 -> [_ w661]
                tunnel: w645 -> [w654 w660]
                tunnel: w618 -> [_ w659]
                tunnel: w617 -> [w655 w658]
                tunnel: [w654 w657] -> w585
                tunnel: [w655 w656] -> w586
                frame False {
                }
                frame True {
                  n134 = Build Array (concatenate) "dT in Array einf."(w658, w659) -> (w656:dbl[])
                  n135 = Build Array (concatenate) "nRolle in Array einf."(w660, w661) -> (w657:dbl[])
                }
              }
              n136 = local read "Differenzenquotient"() -> (w598:u8)
              n137 = case shown="\"Zündsignal\"" w590 {
                tunnel: w647 -> [_ _ w725]
                tunnel: w646 -> [_ _ w724]
                tunnel: [w720 "nKuWe/nRolle" w723] -> w651
                tunnel: w650 -> [w721 _ _]
                frame "Getriebe & Reifen" {
                  n138 = Divide(x=w721, y="Reifenumfang [m]") -> (x/y=w719:dbl)
                  n139 = Multiply(x=w719, y="Getriebe [1:]") -> (x*y=w720:dbl)
                }
                frame "nKuWe / nRolle" {
                }
                frame "Zündsignal" {
                  n140 = Divide(x=w725, y=w724) -> (x/y=w723:dbl)
                }
              }
              n141 = Multiply(x=2, y=w598) -> (x*y=w596:i32)
              n142 = Increment(x=w596) -> (x+1=w594:i32)
              n143 = Index Array(array=w586, index=1 ("Index")) -> (element=w605:dbl)
              n144 = Index Array(array=w585, index=1 ("Index")) -> (element=w611:dbl)
              n145 = Initialize Array(w605, w594) -> (w603:dbl[])
              n146 = Initialize Array(w611, w602) -> (w610:dbl[])
              n147 = Insert Into Array(array=w586, index=0 ("Index"), new element=w603) -> (w601:dbl[])
              n148 = Insert Into Array(array=w585, index=0 ("Index"), new element=w610) -> (w608:dbl[])
              n149 = call-poly <vilib>:"IIR Filter.vi"("Forward Coefficients"=w599, "Reverse Coefficients"=w600, "X"=w601) -> ("Filtered X"=w595:dbl[])  [unwired: 1 in, 1 out]
              n150 = call-poly <vilib>:"IIR Filter.vi"("Forward Coefficients"=w648, "Reverse Coefficients"=w649, "X"=w608) -> ("Filtered X"=w607:dbl[])  [unwired: 1 in, 1 out]
              n151 = case shown="False" w589 {
                selector: w589 -> [_ w716]
                tunnel: w651 -> [w704 _]
                tunnel: w653 -> [w706 w715]
                tunnel: [w701 w716] -> w644
                tunnel: [w705 w715] -> w652
                tunnel: w620 -> [w703 w714]
                tunnel: [w701 w714] -> w619
                tunnel: w590 -> [w700 _]
                frame False {
                  n152 = Build Array (concatenate)(w706, w704) -> (w705:dbl[])
                  n153 = case shown="\"Zündsignal\"" w700 {
                    tunnel: ["Dauer [s]" 0.0 ("Dauer [s]") 0.0] -> w702
                    frame "Zündsignal" {
                      n154 = property on="Untersetzung\nermittelt" class="Bool. (strikt)"("Blinking"=TRUE ("Blinkend"), "BoolText.Text"="Ermittle Übersetzung" ("Boolescher Text.Text")) -> ()  [unwired: 2 in, 2 out]
                    }
                    frame "Getriebe & Reifen", Default {
                    }
                    frame "nKuWe / nRolle" {
                    }
                  }
                  n155 = call "Verstrichene Zeit"("Time Target (s)"=w702, "Reset"=w703) -> ("Time has Elapsed"=w701:bool)  [unwired: 10 in, 7 out]
                  n156 = case shown="True" w701 {
                    frame False {
                    }
                    frame True {
                      n157 = property on="Untersetzung\nermittelt" class="Bool. (strikt)"("Blinking"=FALSE ("Blinkend"), "BoolText.Text"="Go" ("Boolescher Text.Text")) -> ()  [unwired: 2 in, 2 out]
                    }
                  }
                  "Untersetzung-Graph" <- w704
                }
                frame True {
                }
              }
              n158 = Array Subset "dT gefiltert [s]"(array=w595, index=w594) -> (w591:dbl[])  [unwired: 1 in]
              n159 = Array Subset "Rolle gefiltert [1/min]"(array=w607, index=w602) -> (w593:dbl[])  [unwired: 1 in]
              n160 = Array Size "Array-Größe"(array=w593) -> (size(s)=w642:i32)
              n161 = Greater?(x=w642, y=w602) -> (0:w643:bool)
              n162 = Square(x=w621) -> (x^2=w640:dbl)
              n163 = Multiply(x=w593, y=w621) -> (x*y=w627:dbl[])
              n164 = Multiply(x=w627, y=w641) -> (x*y=w592:dbl[])
              n165 = Divide(x="Rollenträgheit [kgm²]", y=w640) -> (x/y=w632:dbl)
              n166 = Multiply(x=w632, y=w631) -> (x*y=w630:dbl)
              n167 = And(x=w644, y=w643) -> (x .and. y?=w613:bool)
              n168 = Array Size "Array-Größe"(array=w592) -> (size(s)=w584:i32)
              n169 = Decrement(x=w584) -> (x-1=w629:i32)
              n170 = Select(t=w615, s=w613, f=1000000.0) -> (s? t:f=w616:dbl)
              n171 = Initialize Array(0.0 ("y"), 0) -> (w635:dbl[])
              n172 = for {
                N: w584 -> [_]
                tunnel: "Differenzenquotient" -> [w676]
                tunnel: w592 -> [w684]
                tunnel: w629 -> [w675]
                shift-right: [w681] -> w628
                shift-left: w635 -> [w682]
                tunnel: w627 -> [w679] mode=indexing
                tunnel: w626 -> [w668]
                tunnel: w616 -> [w678]
                tunnel: [w669] -> w625
                tunnel: w624 -> [w667]
                tunnel: w591 -> [w664] mode=indexing
                i -> [w665]
                stop <- w662 stop-if-true
                n173 = Multiply(x=w664, y=2.0) -> (x*y=w666:dbl)
                n174 = Subtract(x=w675, y=w676) -> (x-y=w677:i32)
                n175 = Subtract(x=w665, y=w676) -> (x-y=w697:i32)
                n176 = Add(x=w665, y=w676) -> (x+y=w691:i32)
                n177 = Greater Or Equal?(x=w665, y=w676) -> (x >= y?=w672:bool)
                n178 = Greater?(x=w679, y=w678) -> (0:w680:bool)
                n179 = Max & Min(x=w675, y=w691) -> (min(x,y)=w692:i32)  [unwired: 1 out]
                n180 = Max & Min(x=w697, y=0) -> (max(x,y)=w695:i32)  [unwired: 1 out]
                n181 = Subtract(x=w692, y=w665) -> (x-y=w693:i32)
                n182 = Less Or Equal?(x=w665, y=w677) -> (x <= y?=w673:bool)
                n183 = Subtract(x=w665, y=w695) -> (x-y=w694:i32)
                n184 = Max & Min(x=w694, y=w693) -> (min(x,y)=w685:i32)  [unwired: 1 out]
                n185 = Add(x=w665, y=w685) -> (x+y=w690:i32)
                n186 = Subtract(x=w665, y=w685) -> (x-y=w689:i32)
                n187 = Multiply(x=w685, y=w666) -> (x*y=w683:dbl)
                n188 = Index Array(array=w684, index=w690) -> (element=w687:dbl)
                n189 = Index Array(array=w684, index=w689) -> (element=w688:dbl)
                n190 = Subtract(x=w687, y=w688) -> (x-y=w686:dbl)
                n191 = Divide(x=w686, y=w683) -> (x/y=w674:dbl)
                n192 = Less Than 0?(x=w674) -> (x < 0?=w671:bool)
                n193 = Less Or Equal To 0?(x=w668) -> (x <= 0?=w670:bool)
                n194 = Build Array (concatenate)(w682, w674) -> (w681:dbl[])
                n195 = Compound Arithmetic op=AND(w671, w680, w670, w672, w673, w667) -> (w662:bool)
                n196 = case shown="False" w662 {
                  tunnel: w665 -> [_ w699]
                  tunnel: [w698 w699] -> w669
                  tunnel: w668 -> [w698 _]
                  frame False {
                  }
                  frame True {
                  }
                }
              }
              n197 = Multiply(x=w628, y=w630) -> (x*y=w639:dbl[])
              n198 = Multiply(x=w592, y=w639) -> (x*y=w633:dbl[])
              n199 = Multiply(x=w634, y=w633) -> (x*y=w638:dbl[])
            }
          }
          "Untersetzung\nermittelt" <- w432
          n200 = local read "Übersetzung ermitteln aus"() -> (w433:T2)
          n201 = Equal To 0? "aus Zündsignal?"(x=w433) -> (x = 0?=w431:bool)
          n202 = case shown="True" w428 {
            tunnel: [FALSE w509] -> w476
            tunnel: w475 -> [_ w508]
            frame False {
            }
            frame True {
              n203 = Greater Than 0?(x=w508) -> (x > 0?=w509:bool)
            }
          }
          n204 = And(x=w432, y=w431) -> (x .and. y?=w430:bool)
          n205 = Select(t=w429, s=w432, f=0.0) -> (s? t:f=→"Untersetzung":dbl)
          n206 = case shown="True" w430 {
            tunnel: w429 -> [_ w510]
            frame False {
            }
            frame True {
              n207 = local write "nKuWe/nRolle"(w510) -> ()
            }
          }
          n208 = local read "Start"() -> (w444:bool)
          n209 = Not(x=w444) -> (.not. x?=w443:bool)
          n210 = Or(x=w476, y=w443) -> (x .or. y?=w479:bool)
        }
        n211 = VISA Clear(VISA resource name=w19, error in (no error)=w18) -> (VISA resource name out=w16:refnum<visa-resource-name>, error out=w20:errorcluster)
        n212 = VISA Close(VISA resource name=w16, error in (no error)=w20) -> ()  [unwired: 1 out]
        n213 = case shown="True" w47 {
          tunnel: w45 -> [_ w406]
          tunnel: w44 -> [_ w411]
          tunnel: w43 -> [_ w410]
          tunnel: w42 -> [_ w382]
          tunnel: w15 -> [_ w407]
          tunnel: w41 -> [_ w405]
          tunnel: w40 -> [_ w399]
          tunnel: w35 -> [_ w385]
          tunnel: ["" w384] -> w36
          tunnel: w37 -> [_ w383]
          tunnel: ["" w381] -> _
          tunnel: [w361 w369] -> _
          frame False {
            w362 = 0.0
            n214 = Initialize Array(w362, w362) -> (w361:dbl[])
          }
          frame True {
            w380 = 0
            n215 = Array Subset "P"(array=w410, length=w382) -> (w402:dbl[])  [unwired: 1 in]
            n216 = Array Subset "n"(array=w406, length=w382) -> (w404:dbl[])  [unwired: 1 in]
            n217 = Array Subset "alpha"(array=w407, length=w382) -> (w408:dbl[])  [unwired: 1 in]
            n218 = Array Subset "M"(array=w411, length=w382) -> (w403:dbl[])  [unwired: 1 in]
            n219 = property on="Pmax" class="Str"("Text.FontSize"=48) -> ()  [unwired: 2 in, 2 out]
            n220 = property on="Ergebnis" class="Str"("Text.FontSize"=18) -> ()  [unwired: 2 in, 2 out]
            n221 = Array Size(array=w408) -> (size(s)=w409:i32)
            n222 = for {
              N: w409 -> [w427]
              tunnel: w407 -> [w424]
              tunnel: w406 -> [w421]
              tunnel: w405 -> [w418]
              tunnel: [w416] -> w379
              i -> [w422]
              stop <- w417 stop-if-true
              n223 = Decrement(x=w427) -> (x-1=w426:i32)
              n224 = Subtract(x=w426, y=w422) -> (x-y=w416:i32)
              n225 = Index Array(array=w421, index=w416) -> (element=w420:dbl)
              n226 = Index Array(array=w424, index=w416) -> (element=w425:dbl)
              n227 = Less?(x=w420, y=w418) -> (x < y?=w419:bool)
              n228 = Less Or Equal To 0?(x=w425) -> (x <= 0?=w423:bool)
              n229 = And(x=w423, y=w419) -> (x .and. y?=w417:bool)
            }
            n230 = Increment(x=w379) -> (x+1=w378:i32)
            n231 = Array Subset "P"(array=w402, index=w378) -> (w370:dbl[])  [unwired: 1 in]
            n232 = Array Subset "n"(array=w404, index=w378) -> (w375:dbl[])  [unwired: 1 in]
            n233 = Array Subset "M"(array=w403, index=w378) -> (w369:dbl[])  [unwired: 1 in]
            n234 = Array Max & Min "nmax [1/min]"(array=w375) -> (max value=w401:dbl)  [unwired: 3 out]
            n235 = Array Max & Min "Mmax"(array=w369) -> (max value=w376:dbl, max index (indices)=w372:i32)  [unwired: 2 out]
            n236 = Bundle(w375, w370) -> (w374:cluster{dbl[], dbl[]})  [unwired: 1 in]
            n237 = Bundle(w375, w369) -> (w373:cluster{dbl[], dbl[]})  [unwired: 1 in]
            n238 = Array Max & Min "Pmax"(array=w370) -> (max value=w377:dbl, max index (indices)=w371:i32)  [unwired: 2 out]
            n239 = Index Array "n(Mmax)"(array=w375, index=w372) -> (element=w392:dbl)
            n240 = Index Array "n(Pmax)"(array=w375, index=w371) -> (element=w397:dbl)
            n241 = Multiply(x=w377, y=1.2) -> (x*y=w366:dbl)
            n242 = Multiply(x=w376, y=1.8) -> (x*y=w367:dbl)
            n243 = Divide(x=w401, y=w383) -> (x/y=w400:dbl)
            n244 = Round To Nearest(number=w366) -> (nearest integer value=w365:dbl)
            n245 = Round To Nearest(number=w367) -> (nearest integer value=w368:dbl)
            n246 = Format Into String(format string="%.1f PS" ("Format-String"), w377) -> (resulting string=→"Pmax":string)  [unwired: 2 in, 1 out]
            n247 = Build Array(w374, w373) -> (→"XY-Graph":cluster{dbl[], dbl[]}[])
            n248 = local read "Lufttemperatur [°C]"() -> (w394:dbl)
            n249 = local read "Luftfeuchtigkeit [%]"() -> (w395:dbl)
            n250 = property on="XY-Graph" class="XYGraph (strikt)"("ActYScl"=w380, "YScale.Maximum"=w365, "YScale.Minimum"=w380) -> ()  [unwired: 2 in, 2 out]
            n251 = local read "Luftdruck [mbar]"() -> (w396:dbl)
            n252 = property on="XY-Graph" class="XYGraph (strikt)"("ActYScl"=1, "YScale.Maximum"=w368, "YScale.Minimum"=w380) -> ()  [unwired: 2 in, 2 out]
            n253 = Compound Arithmetic op=MULTIPLY "vmax"(w400, w399, 0.06) -> (w391:dbl)
            n254 = Format Date/Time String(time format string (%c)="%x %H:%M ") -> (date/time string=w384:string)  [unwired: 2 in]
            n255 = Format Into String(format string="%.1f PS bei %d 1/min   |   %.1f Nm bei %d 1/min   |   vmax: %d km/h\\nDIN 70020 k =%.3f (%d \\B0C, %d %%, %d mbar)\\n%s" ("Format-String"), w377, w397, w376, w392, w391, w385, w394, w395, w396, w384) -> (resulting string=w381:string)  [unwired: 2 in, 1 out]
            "Ergebnis" <- w381
          }
        }
        n256 = flat-sequence {
          tunnel: w29 -> [w324]
          tunnel: w31 -> [w325]
          tunnel: w34 -> [w326]
          tunnel: w35 -> [w327]
          tunnel: w36 -> [w328]
          tunnel: w37 -> [w329]
          tunnel: w38 -> [w330]
          tunnel: w39 -> [w331]
          tunnel: [w331] -> w131
          tunnel: [w330] -> w130
          tunnel: [w329] -> w129
          tunnel: [w328] -> w128
          tunnel: [w327] -> w127
          tunnel: [w326] -> w126
          tunnel: [w325] -> w125
          tunnel: [w324] -> w124
          tunnel: [w320] -> w17
          tunnel: w16 -> [w320]
          tunnel: w131 -> [w360]
          tunnel: w130 -> [w359]
          tunnel: w129 -> [w358]
          tunnel: w128 -> [w357]
          tunnel: w127 -> [w356]
          tunnel: w126 -> [w355]
          tunnel: w125 -> [w354]
          tunnel: w124 -> [w353]
          tunnel: w17 -> [w335]
          frame #0 {
            w322 = FALSE ("Start [F1]")
            w323 = 0  # Aktivieren
            n257 = local write "Start"(w322) -> ()
            n258 = property on="Speichern" class="Bool. (strikt)"("DisabledEnum"=w323) -> ()  [unwired: 2 in, 2 out]
            n259 = property on="Übersetzung ermitteln aus" class="Enum (strikt)"("DisabledEnum"=w323) -> ()  [unwired: 2 in, 2 out]
            n260 = property on="Konfiguration:" class="Bool. (strikt)"("DisabledEnum"=w323) -> ()  [unwired: 2 in, 2 out]
            n261 = property on="Ende" class="Bool. (strikt)"("DisabledEnum"=w323) -> ()  [unwired: 2 in, 2 out]
            n262 = property on="Drucken" class="Bool. (strikt)"("DisabledEnum"=w323) -> ()  [unwired: 2 in, 2 out]
            n263 = property on="Untersetzung\nermittelt" class="Bool. (strikt)"("BoolText.Text"="GO" ("Boolescher Text.Text"), "Blinking"=w322) -> ()  [unwired: 2 in, 2 out]
            n264 = local write "Untersetzung\nermittelt"(w322) -> ()
          }
          frame #1 {
            w332 = dbl[] []
            w338 = 0.0
            n265 = local read "Übersetzung ermitteln aus"() -> (w341:T2)
            n266 = local read "Rollenträgheit [kgm²]"() -> (w350:dbl)
            n267 = local read "Gleitender Mittelwert"() -> (w346:u8)
            n268 = local read "Messung Klimadaten"() -> (w337:bool)
            n269 = local read "Rollengeber [Inkr/U]"() -> (w351:u16)
            n270 = local read "Lufttemperatur [°C]"() -> (w344:dbl)
            n271 = local read "Differenzenquotient"() -> (w345:u8)
            n272 = local read "Luftfeuchtigkeit [%]"() -> (w343:dbl)
            n273 = local read "Reifenumfang [m]"() -> (w347:dbl)
            n274 = local read "n vom Gas [1/min]"() -> (w339:dbl)
            n275 = local read "Zündung [Imp/U]"() -> (w349:dbl)
            n276 = local read "Luftdruck [mbar]"() -> (w342:dbl)
            n277 = local read "nKuWe/nRolle"() -> (w334:dbl)
            n278 = local read "Getriebe [1:]"() -> (w348:dbl)
            n279 = local read "Dauer [s]"() -> (w340:dbl)
            n280 = Bundle("Fahrzeugdaten"="Fahrzeugdaten", "date/time string"=w357, "Rollengeber [Inkr/U]"=w351, "Rollenumfang [m]"=w355, "Rollenträgheit [kgm²]"=w350, "Zündung [Imp/U]"=w349, "Getriebe [1:]"=w348, "Reifenumfang [m]"=w347, "mean value"=w358, "Gleitender Mittelwert"=w346, "Differenzenquotient"=w345, 0, w360, "element"=w356, "Lufttemperatur [°C]"=w344, "Luftfeuchtigkeit [%]"=w343, "Luftdruck [mbar]"=w342, w359, w332, w332, w332, "Übersetzung ermitteln aus"=w341, "Dauer [s]"=w340, w338, w338, "n vom Gas [1/min]"=w339, w354, w353, "Messung Klimadaten"=w337, "VISA resource name out"=w335, "nKuWe/nRolle"=w334) -> (→"Datenspeicher":T5)  [unwired: 1 in]
          }
        }
      }
    }
    n281 = local read "Ende"() -> (w1:bool)
  }
  n282 = flat-sequence {
    frame #0 {
      n283 = call <vilib>:"Application Directory.vi"() -> ("Application Directory"=w842:path)
      n284 = Build Path(base path=w842, name or relative path="Konfig.xml") -> (appended path=w840:path)
      n285 = call-poly <vilib>:"Read From XML File.vi"("XML File Path"=w840) -> ("error out"=w822:errorcluster, "XML Elements"=w844:string)  [unwired: 8 in, 1 out]
      n286 = property on="Datenspeicher" class="Cluster (strikt)"() -> ("Value"=w843:T3)  [unwired: 2 in, 2 out]
      n287 = case shown="Kein Fehler" w822 {
        tunnel: w844 -> [w847 _]
        tunnel: w843 -> [w846 _]
        tunnel: [w845 T6 {"Fahrzeugdaten"="", "date/time string"="05.02.2017 22:14 ", "Rolle [Inkr/U]"=10, "Rollenumfang [m]"=0.613, "Rollenträgheit [kgm²]"=0.402, "Zündung [Imp/U]"=5.0, "Getriebe [1:]"=5.343, "Reifenumfang [m] "=1.222, "element"=2.0, "Gl. Mittelwert"=35, "Differenzenquotient"=12, "Polynom"=15, "element"=0.01639344262295082, "element"=1.0177230216140456, "Lufttemperatur [°C]"=23.3, "Luftfeuchtigkeit [%]"=43.8, "Luftdruck [mbar]"=1013.45, array[1238 elements], array[1224 elements], "Best Polynomial Fit"=array[1224 elements], array[1224 elements], "Übersetzung ermitteln aus"=0, "[s]"=5.0, "nmin [1/min]"=0.0, "nmax [1/min]"=0.0, "n vom Gas [1/min]"=5000.0, array[1238 elements], array[1238 elements], "Boolesch"=TRUE, "Serielle Schnittstelle"="", 10.0} ("Datenspeicher")] -> w823
        frame No Error {
          n288 = Unflatten From XML(xml string=w847, type=w846) -> (value=w845:T3)  [unwired: 1 in, 1 out]
        }
        frame Error {
        }
      }
      n289 = property on="Datenspeicher" class="Cluster (strikt)"("Value"=w823) -> ()  [unwired: 2 in, 2 out]
      n290 = Unbundle(w823) -> ("Fahrzeugdaten"=w839:string, "Rolle [Inkr/U]"=w838:u16, "Rollenumfang [m]"=w837:dbl, "Rollenträgheit [kgm²]"=w836:dbl, "Zündung [Imp/U]"=w835:dbl, "Getriebe [1:]"=w834:dbl, "Reifenumfang [m]"=w833:dbl, "element"=w821:dbl, "Gl. Mittelwert"=w832:u8, "Differenzenquotient"=w831:u8, "Lufttemperatur [°C]"=w830:dbl, "Luftfeuchtigkeit [%]"=w829:dbl, "Luftdruck [mbar]"=w828:dbl, "Übersetzung ermitteln aus"=w825:u8, "[s]"=w827:dbl, "n vom Gas [1/min]"=w826:dbl, "Boolesch"=w824:bool, "Serielle Schnittstelle"=w820:refnum<visa-resource-name>, "nKuWe/nRolle"=w819:dbl)  [unwired: 12 out]
      n291 = property on="Dauer [s]" class="DigWert (strikt)"("Value"=w827) -> ()  [unwired: 2 in, 2 out]
      n292 = property on="Fahrzeugdaten" class="Str"("Value"=w839) -> ()  [unwired: 2 in, 2 out]
      n293 = property on="Rollengeber [Inkr/U]" class="DigWert (strikt)"("Value"=w838) -> ()  [unwired: 2 in, 2 out]
      n294 = property on="Rollenumfang [m]" class="DigWert (strikt)"("Value"=w837) -> ()  [unwired: 2 in, 2 out]
      n295 = property on="Rollenträgheit [kgm²]" class="DigWert (strikt)"("Value"=w836) -> ()  [unwired: 2 in, 2 out]
      n296 = property on="Zündung [Imp/U]" class="DigWert (strikt)"("Value"=w835) -> ()  [unwired: 2 in, 2 out]
      n297 = property on="Getriebe [1:]" class="DigWert (strikt)"("Value"=w834) -> ()  [unwired: 2 in, 2 out]
      n298 = property on="Reifenumfang [m]" class="DigWert (strikt)"("Value"=w833) -> ()  [unwired: 2 in, 2 out]
      n299 = property on="nKuWe/nRolle" class="DigWert (strikt)"("Value"=w821) -> ()  [unwired: 2 in, 2 out]
      n300 = property on="Gleitender Mittelwert" class="DigWert (strikt)"("Value"=w832) -> ()  [unwired: 2 in, 2 out]
      n301 = property on="Differenzenquotient" class="DigWert (strikt)"("Value"=w831) -> ()  [unwired: 2 in, 2 out]
      n302 = property on="Lufttemperatur [°C]" class="DigWert (strikt)"("Value"=w830) -> ()  [unwired: 2 in, 2 out]
      n303 = property on="Luftfeuchtigkeit [%]" class="DigWert (strikt)"("Value"=w829) -> ()  [unwired: 2 in, 2 out]
      n304 = property on="Luftdruck [mbar]" class="DigWert (strikt)"("Value"=w828) -> ()  [unwired: 2 in, 2 out]
      n305 = property on="Übersetzung ermitteln aus" class="Enum (strikt)"("Val(Sgnl)"=w825) -> ()  [unwired: 2 in, 2 out]
      n306 = property on="n vom Gas [1/min]" class="DigWert (strikt)"("Value"=w826) -> ()  [unwired: 2 in, 2 out]
      n307 = property on="Messung Klimadaten" class="Bool. (strikt)"("Val(Sgnl)"=w824) -> ()  [unwired: 2 in, 2 out]
      n308 = local write "Serielle Schnittstelle"(w820) -> ()
      n309 = property on="nKuWe/nRolle" class="DigWert (strikt)"("Value"=w819) -> ()  [unwired: 2 in, 2 out]
    }
    frame #1 {
      w855 = 2  # Deaktivieren
      w857 = 0.0  # Graphen löschen
      n310 = local read "Serielle Schnittstelle"() -> (w853:refnum<visa-resource-name>)
      n311 = property on="Frontpanel-Position" class="Bereich"("Origin"=T7 {"Horizontal"=8, "Vertical"=6}) -> ()  [unwired: 2 in, 2 out]
      n312 = property on="Füllstand Lesepuffer" class="Schieber (strikt)"("Scale.Maximum"=100) -> ()  [unwired: 2 in, 2 out]
      n313 = property on="Drucken" class="Bool. (strikt)"("DisabledEnum"=w855) -> ()  [unwired: 2 in, 2 out]
      n314 = property on="Speichern" class="Bool. (strikt)"("DisabledEnum"=w855) -> ()  [unwired: 2 in, 2 out]
      n315 = Build Array(w857) -> (w856:dbl[])
      n316 = VISA Clear(VISA resource name=w853) -> (VISA resource name out=w852:refnum<visa-resource-name>, error out=w851:errorcluster)  [unwired: 1 in]
      n317 = property on="Untersetzung-Graph" class="SVDiagr (strikt)"("History Data"=w856) -> ()  [unwired: 2 in, 2 out]
      n318 = VISA Close(VISA resource name=w852, error in (no error)=w851) -> (error out=w850:errorcluster)
      n319 = case shown="Kein Fehler" w850 {
        tunnel: [T4."Enabled" ("Deaktiviert") T4."Disabled and Grayed Out" ("Deaktiviert")] -> w849
        frame No Error {
        }
        frame Error {
        }
      }
      n320 = property on="Start" class="Bool. (strikt)"("DisabledEnum"=w849) -> ()  [unwired: 2 in, 2 out]
    }
  }
  n321 = while {
    stop <- w861 stop-if-true
    n322 = event shown="[4] \"Leistung\": Wertänderung" {
      selector: _ -> [_ _ _ _ _ _ _ _ _]
      dyn-events: _ -> [_ _ _ _ _ _ _ _ _]
      timeout: _ -> [_ _ _ _ _ _ _ _ _]
      tunnel: [_ _ _ TRUE _ _ _ _ _] -> w861
      event "Konfiguration:": Value Change {
        n323 = event-data() -> ("OldVal"=w863:bool)  [unwired: 1 in, 5 out]
        n324 = flat-sequence {
          tunnel: [w867] -> w864
          tunnel: w863 -> [w867]
          tunnel: w864 -> [w893]
          frame #0 {
            n325 = call-poly <vilib>:"Read From XML File.vi"() -> ("error out"=w865:errorcluster, "XML Elements"=w868:string)  [unwired: 9 in, 1 out]
            n326 = property on="Datenspeicher" class="Cluster (strikt)"() -> ("Value"=w866:T3)  [unwired: 2 in, 2 out]
            n327 = case shown="Kein Fehler" w865 {
              selector: w865 -> [_ w892]
              tunnel: w868 -> [w872 _]
              tunnel: w866 -> [w871 _]
              frame No Error {
                n328 = Unflatten From XML(xml string=w872, type=w871) -> (value=w870:T3, error out=w869:errorcluster)  [unwired: 1 in]
                n329 = case shown="Kein Fehler" w869 {
                  tunnel: w870 -> [w890 _]
                  frame No Error {
                    n330 = Unbundle(w890) -> ("Fahrzeugdaten"=w889:string, "Rolle [Inkr/U]"=w888:u16, "Rollenumfang [m]"=w887:dbl, "Rollenträgheit [kgm²]"=w886:dbl, "Zündung [Imp/U]"=w885:dbl, "Getriebe [1:]"=w884:dbl, "Reifenumfang [m]"=w883:dbl, "Gl. Mittelwert"=w882:u8, "Differenzenquotient"=w881:u8, "Lufttemperatur [°C]"=w880:dbl, "Luftfeuchtigkeit [%]"=w879:dbl, "Luftdruck [mbar]"=w878:dbl, "Übersetzung ermitteln aus"=w875:u8, "[s]"=w877:dbl, "n vom Gas [1/min]"=w876:dbl, "Boolesch"=w874:bool, "nKuWe/nRolle"=w873:dbl)  [unwired: 14 out]
                    n331 = property on="Dauer [s]" class="DigWert (strikt)"("Value"=w877) -> ()  [unwired: 2 in, 2 out]
                    n332 = property on="Fahrzeugdaten" class="Str"("Value"=w889) -> ()  [unwired: 2 in, 2 out]
                    n333 = property on="Rollengeber [Inkr/U]" class="DigWert (strikt)"("Value"=w888) -> ()  [unwired: 2 in, 2 out]
                    n334 = property on="Rollenumfang [m]" class="DigWert (strikt)"("Value"=w887) -> ()  [unwired: 2 in, 2 out]
                    n335 = property on="Rollenträgheit [kgm²]" class="DigWert (strikt)"("Value"=w886) -> ()  [unwired: 2 in, 2 out]
                    n336 = property on="Zündung [Imp/U]" class="DigWert (strikt)"("Value"=w885) -> ()  [unwired: 2 in, 2 out]
                    n337 = property on="Getriebe [1:]" class="DigWert (strikt)"("Value"=w884) -> ()  [unwired: 2 in, 2 out]
                    n338 = property on="Reifenumfang [m]" class="DigWert (strikt)"("Value"=w883) -> ()  [unwired: 2 in, 2 out]
                    n339 = property on="Gleitender Mittelwert" class="DigWert (strikt)"("Value"=w882) -> ()  [unwired: 2 in, 2 out]
                    n340 = property on="Differenzenquotient" class="DigWert (strikt)"("Value"=w881) -> ()  [unwired: 2 in, 2 out]
                    n341 = property on="Lufttemperatur [°C]" class="DigWert (strikt)"("Value"=w880) -> ()  [unwired: 2 in, 2 out]
                    n342 = property on="Luftfeuchtigkeit [%]" class="DigWert (strikt)"("Value"=w879) -> ()  [unwired: 2 in, 2 out]
                    n343 = property on="Luftdruck [mbar]" class="DigWert (strikt)"("Value"=w878) -> ()  [unwired: 2 in, 2 out]
                    n344 = property on="Übersetzung ermitteln aus" class="Enum (strikt)"("Val(Sgnl)"=w875) -> ()  [unwired: 2 in, 2 out]
                    n345 = property on="n vom Gas [1/min]" class="DigWert (strikt)"("Value"=w876) -> ()  [unwired: 2 in, 2 out]
                    n346 = property on="Messung Klimadaten" class="Bool. (strikt)"("Val(Sgnl)"=w874) -> ()  [unwired: 2 in, 2 out]
                    n347 = property on="nKuWe/nRolle" class="DigWert (strikt)"("Value"=w873) -> ()  [unwired: 2 in, 2 out]
                  }
                  frame Error {
                    n348 = One Button Dialog(message="Dateiversion nicht kompatibel" ("Nachricht")) -> ()  [unwired: 1 in, 1 out]
                  }
                }
              }
              frame Error {
                n349 = call <vilib>:"Clear Errors.vi"("error in (no error)"=w892) -> ()  [unwired: 5 in, 2 out]
              }
            }
          }
          frame #1 {
            n350 = property on="Konfiguration:" class="Bool. (strikt)"("Value"=w893) -> ()  [unwired: 2 in, 2 out]
          }
        }
      }
      event "Drucken": Value Change {
        n351 = event-data() -> ("OldVal"=w894:bool)  [unwired: 1 in, 5 out]
        n352 = flat-sequence {
          tunnel: [w899] -> w895
          tunnel: w894 -> [w899]
          tunnel: w895 -> [w900]
          frame #0 {
            n353 = control-ref of="Fahrzeugdaten"() -> (w897:refnum<vi>)
            n354 = control-ref of="XY-Graph"() -> (w898:refnum<vi>)
            n355 = control-ref of="Ergebnis"() -> (w896:refnum<vi>)
            n356 = call "printgraph_V0.01.vi"("reference 2"=w896, "Fahrzeugdaten"=w897, "XYGraph (Eingang)"=w898) -> ()  [unwired: 9 in]
          }
          frame #1 {
            n357 = property on="Drucken" class="Bool. (strikt)"("Value"=w900) -> ()  [unwired: 2 in, 2 out]
          }
        }
      }
      event "Speichern": Value Change {
        n358 = event-data() -> ("OldVal"=w902:bool)  [unwired: 1 in, 5 out]
        n359 = call <vilib>:"Three Button Dialog.vi"("Center Button Text (\"No\")"="Excel" ("Text für F-Schaltfläche (\"Abbrechen\")"), "Left Button Text (\"Yes\")"="ReCalc" ("Text für T-Schaltfläche (\"OK\")"), "message"="Welches Format soll gespeichert werden?" ("Nachricht")) -> ("Which Button?"=w903:T10)  [unwired: 8 in]
        n360 = case shown="\"Center Button\"" w903 {
          tunnel: w902 -> [w907 w909]
          tunnel: [w907 w909] -> w901
          frame "Left Button", Default {
            n361 = control-ref of="Datenspeicher"() -> (w908:refnum<vi>)
            n362 = call "savecluster_V0.01.vi"("Datenspeicher 3"=w908) -> ()  [unwired: 2 in]
          }
          frame "Center Button" {
            n363 = invoke on="XY-Graph" class="XYGraph (strikt)" method="Daten in Excel exportieren"() -> ()  [unwired: 3 in, 3 out]
          }
        }
        n364 = local write "Speichern"(w901) -> ()
      }
      event "Ende": Value Change {
        w913 = 0.0 ("element")
        (unwired) 0.0 ("element")
        n365 = event-data() -> ("OldVal"=w911:bool)  [unwired: 1 in, 5 out]
        n366 = flat-sequence {
          tunnel: w911 -> [w945]
          tunnel: [w945] -> w910
          frame #0 {
            n367 = Wait (ms)(milliseconds to wait=u32 100 ("Zu wartende ms")) -> ()  [unwired: 1 out]
          }
        }
        n368 = local read "Datenspeicher"() -> (w914:T3)
        n369 = Unbundle By Name(w914) -> ("Rolle [Inkr/U]"=w935:u16, "Rollenumfang [m]"=w934:dbl, "Rollenträgheit [kgm²]"=w933:dbl, "Zündung [Imp/U]"=w932:dbl, "Getriebe [1:]"=w931:dbl, "Reifenumfang [m]"=w930:dbl, "Gl. Mittelwert"=w929:u8, "Differenzenquotient"=w928:u8, "Polynom"=w927:u8, "Lufttemperatur [°C]"=w926:dbl, "Luftfeuchtigkeit [%]"=w925:dbl, "Luftdruck [mbar]"=w923:dbl, "Best Polynomial Fit"=w924:dbl[], "Übersetzung ermitteln aus"=w922:u8, "[s]"=w921:dbl, "nmin [1/min]"=w920:dbl, "nmax [1/min]"=w919:dbl, "n vom Gas [1/min]"=w918:dbl, "Boolesch"=w917:bool, "Serielle Schnittstelle"=w912:refnum<visa-resource-name>)  [unwired: 3 out]
        n370 = call <vilib>:"Application Directory.vi"() -> ("Application Directory"=w940:path)
        n371 = local write "Ende"(w910) -> ()
        n372 = Bundle By Name(cluster=w914, "Fahrzeugdaten"="", "date/time string"="", "Rolle [Inkr/U]"=w935, "Rollenumfang [m]"=w934, "Rollenträgheit [kgm²]"=w933, "Zündung [Imp/U]"=w932, "Getriebe [1:]"=w931, "Reifenumfang [m]"=w930, "element"=0.0, "Gl. Mittelwert"=w929, "Differenzenquotient"=w928, "Polynom"=w927, "element"=w913, "element"=w913, "Lufttemperatur [°C]"=w926, "Luftfeuchtigkeit [%]"=w925, "Luftdruck [mbar]"=w923, "Best Polynomial Fit"=w924, "Übersetzung ermitteln aus"=w922, "[s]"=w921, "nmin [1/min]"=w920, "nmax [1/min]"=w919, "n vom Gas [1/min]"=w918, "Boolesch"=w917, "Serielle Schnittstelle"=w912) -> (w915:T3)
        n373 = Build Path(base path=w940, name or relative path="Konfig.xml") -> (appended path=w938:path)
        n374 = Flatten To XML(anything=w915) -> (xml string=w942:string)
        n375 = call-poly <vilib>:"Write to XML File.vi"("XML Input"=w942, "XML File Path"=w938) -> ("error out"=w941:errorcluster)  [unwired: 7 in, 2 out]
        n376 = case shown="Kein Fehler" w941 {
          frame No Error {
          }
          frame Error {
          }
        }
      }
      event "Leistung": Value Change {
        n377 = event-data() -> ("NewVal"=w954:bool)  [unwired: 1 in, 5 out]
        n378 = flat-sequence {
          tunnel: w954 -> [w961]
          tunnel: [w959] -> w953
          tunnel: [w957] -> w952
          tunnel: [w958] -> w951
          tunnel: [w957] -> w950
          tunnel: [w956] -> w948
          tunnel: [w955] -> w946
          tunnel: w953 -> [w981]
          tunnel: w952 -> [w980]
          tunnel: w951 -> [w979]
          tunnel: w950 -> [w978]
          tunnel: [w976] -> w949
          tunnel: w948 -> [w976]
          tunnel: [w975] -> w947
          tunnel: w946 -> [w975]
          tunnel: w949 -> [w983]
          tunnel: w947 -> [w982]
          frame #0 {
            n379 = case shown="True" w961 {
              tunnel: [T9 {"Width"=492, "Height"=492} ("Objektrahmengröße") T9 {"Width"=252, "Height"=252} ("Objektrahmengröße 2")] -> w957
              tunnel: [T8 {"Left"=751, "Top"=246} ("Position") T8 {"Left"=264, "Top"=504} ("Position 2")] -> w958
              tunnel: [T8 {"Left"=258, "Top"=246} ("Position 3") T8 {"Left"=264, "Top"=242} ("Position 4")] -> w959
              tunnel: [FALSE ("Sichtbar") TRUE ("Sichtbar")] -> w960
              tunnel: [T8 {"Left"=955, "Top"=650} ("Position 2") T8 {"Left"=346, "Top"=675} ("Position 2")] -> w956
              tunnel: [T8 {"Left"=462, "Top"=650} ("Position") T8 {"Left"=346, "Top"=410} ("Position")] -> w955
              frame False {
              }
              frame True {
              }
            }
            n380 = property on="XY-Graph" class="XYGraph (strikt)"("Visible"=w960) -> ()  [unwired: 2 in, 2 out]
            n381 = property on="Ergebnis" class="Str"("Visible"=w960) -> ()  [unwired: 2 in, 2 out]
            n382 = property on="Pmax" class="Str"("Visible"=w960) -> ()  [unwired: 2 in, 2 out]
            n383 = property on="Speichern" class="Bool. (strikt)"("Visible"=w960) -> ()  [unwired: 2 in, 2 out]
            n384 = property on="Drucken" class="Bool. (strikt)"("Visible"=w960) -> ()  [unwired: 2 in, 2 out]
            n385 = property on="Fahrzeugdaten" class="Str"("Visible"=w960) -> ()  [unwired: 2 in, 2 out]
          }
          frame #1 {
            n386 = property on="Hinterrad\n[km/h]" class="Drehknopf (strikt)"("Position"=w979, "Housing Size"=w978, "Scale.Increment"=5.0 ("Wertebereich:Inkrement")) -> ()  [unwired: 2 in, 2 out]
            n387 = property on="Welle\n[1/min]" class="Drehknopf (strikt)"("Position"=w981, "Housing Size"=w980) -> ()  [unwired: 2 in, 2 out]
            n388 = Wait (ms)(milliseconds to wait=u32 10 ("Zu wartende ms")) -> ()  [unwired: 1 out]
          }
          frame #2 {
            n389 = property class="DigWert (strikt)" props=["Position", "Bounds"]("Position"=w982) -> ()  [unwired: 2 in, 3 out]
            n390 = property class="DigWert (strikt)"("Position"=w983) -> ()  [unwired: 2 in, 2 out]
          }
        }
      }
      event "Serielle Schnittstelle": Value Change {
        n391 = event-data() -> ()  [unwired: 1 in, 6 out]
        n392 = property on="Start" class="Bool. (strikt)"("DisabledEnum"=T4."Enabled" ("Deaktiviert")) -> ()  [unwired: 2 in, 2 out]
      }
      event "Messung Klimadaten": Value Change {
        n393 = event-data() -> ("NewVal"=w985:bool)  [unwired: 1 in, 5 out]
        n394 = case shown="True" w985 {
          frame True {
            w986 = T4."Disabled and Grayed Out" ("Deaktiviert")
            n395 = property on="Lufttemperatur [°C]" class="DigWert (strikt)"("DisabledEnum"=w986) -> ()  [unwired: 2 in, 2 out]
            n396 = property on="Luftdruck [mbar]" class="DigWert (strikt)"("DisabledEnum"=w986) -> ()  [unwired: 2 in, 2 out]
            n397 = property on="Luftfeuchtigkeit [%]" class="DigWert (strikt)"("DisabledEnum"=w986) -> ()  [unwired: 2 in, 2 out]
          }
          frame False {
            w987 = T4."Enabled" ("Deaktiviert")
            n398 = property on="Lufttemperatur [°C]" class="DigWert (strikt)"("DisabledEnum"=w987) -> ()  [unwired: 2 in, 2 out]
            n399 = property on="Luftdruck [mbar]" class="DigWert (strikt)"("DisabledEnum"=w987) -> ()  [unwired: 2 in, 2 out]
            n400 = property on="Luftfeuchtigkeit [%]" class="DigWert (strikt)"("DisabledEnum"=w987) -> ()  [unwired: 2 in, 2 out]
          }
        }
      }
      event "Recalc": Value Change {
        n401 = event-data() -> ("OldVal"=w990:bool)  [unwired: 1 in, 5 out]
        n402 = property on="Recalc" class="Bool. (strikt)"("Value"=w990) -> ()  [unwired: 2 in, 2 out]
        n403 = property on="Datenspeicher" class="Cluster (strikt)"() -> ("Value"=w988:T3)  [unwired: 2 in, 2 out]
        n404 = call "ReCalc_V2.00.vi"("Berechnen"=TRUE, "Datenspeicher"=w988) -> ()  [unwired: 3 in]
      }
      event "Übersetzung ermitteln aus": Value Change {
        n405 = event-data() -> ("NewVal"=w992:T2)  [unwired: 1 in, 5 out]
        n406 = case shown="\"nKuWe / nRolle\"" w992 {
          tunnel: [T4."Disabled and Grayed Out" ("Deaktiviert") T4."Disabled and Grayed Out" ("Deaktiviert") T4."Enabled" ("Deaktiviert")] -> w994
          frame "nKuWe / nRolle" {
          }
          frame "Zündsignal", Default {
          }
          frame "Getriebe & Reifen" {
          }
        }
        n407 = case shown="\"Zündsignal\", Standard" w992 {
          tunnel: [T4."Enabled" ("Deaktiviert") T4."Disabled and Grayed Out" ("Deaktiviert") T4."Disabled and Grayed Out" ("Deaktiviert")] -> w993
          frame "nKuWe / nRolle" {
          }
          frame "Zündsignal", Default {
          }
          frame "Getriebe & Reifen" {
          }
        }
        n408 = case shown="\"Zündsignal\", Standard" w992 {
          tunnel: [T4."Disabled and Grayed Out" ("Deaktiviert") T4."Enabled" ("Deaktiviert") T4."Disabled and Grayed Out" ("Deaktiviert")] -> w991
          frame "nKuWe / nRolle" {
          }
          frame "Zündsignal", Default {
          }
          frame "Getriebe & Reifen" {
          }
        }
        n409 = property on="Getriebe [1:]" class="DigWert (strikt)"("DisabledEnum"=w994) -> ()  [unwired: 2 in, 2 out]
        n410 = property on="Reifenumfang [m]" class="DigWert (strikt)"("DisabledEnum"=w994) -> ()  [unwired: 2 in, 2 out]
        n411 = property on="nKuWe/nRolle" class="DigWert (strikt)"("DisabledEnum"=w993) -> ()  [unwired: 2 in, 2 out]
        n412 = property on="Dauer [s]" class="DigWert (strikt)"("DisabledEnum"=w991) -> ()  [unwired: 2 in, 2 out]
        n413 = property on="Zündung [Imp/U]" class="DigWert (strikt)"("DisabledEnum"=w991) -> ()  [unwired: 2 in, 2 out]
      }
    }
    n414 = disable-structure shown="Deaktiviert" {
      disable-tunnel: w861 -> [w862 _]
      frame Disabled {
        n415 = Quit LabVIEW(quit? (T)=w862) -> ()
      }
      frame Enabled {
      }
    }
  }
